vi "Write Channel to Text Log File (Waveform).vi"(6 "Waveform Data":waveform(dbl), 8 "error in (no error)":errorcluster, 9 "Channel Name in":string, 10 "Group Name in":string, 11 "Text Log File in":refnum<class "Text Log File.lvclass">) -> (0 "error out":errorcluster, 3 "Text Log File out":refnum<class "Text Log File.lvclass">)   [LabVIEW 2015, in "Text Log File.lvclass"]
uses:
  Text Log File.lvclass
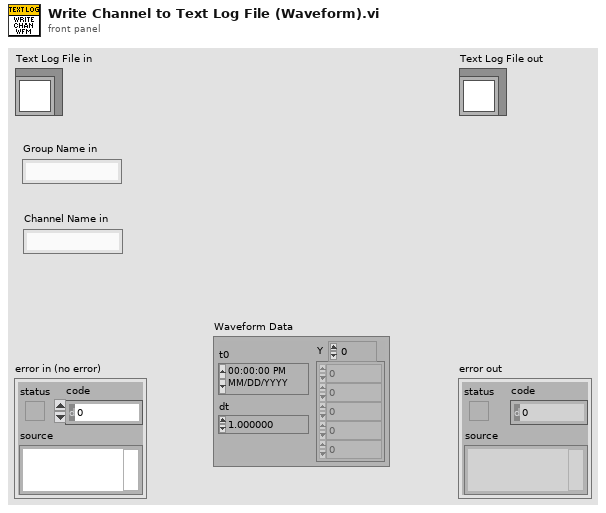
[diagram p1: front panel]
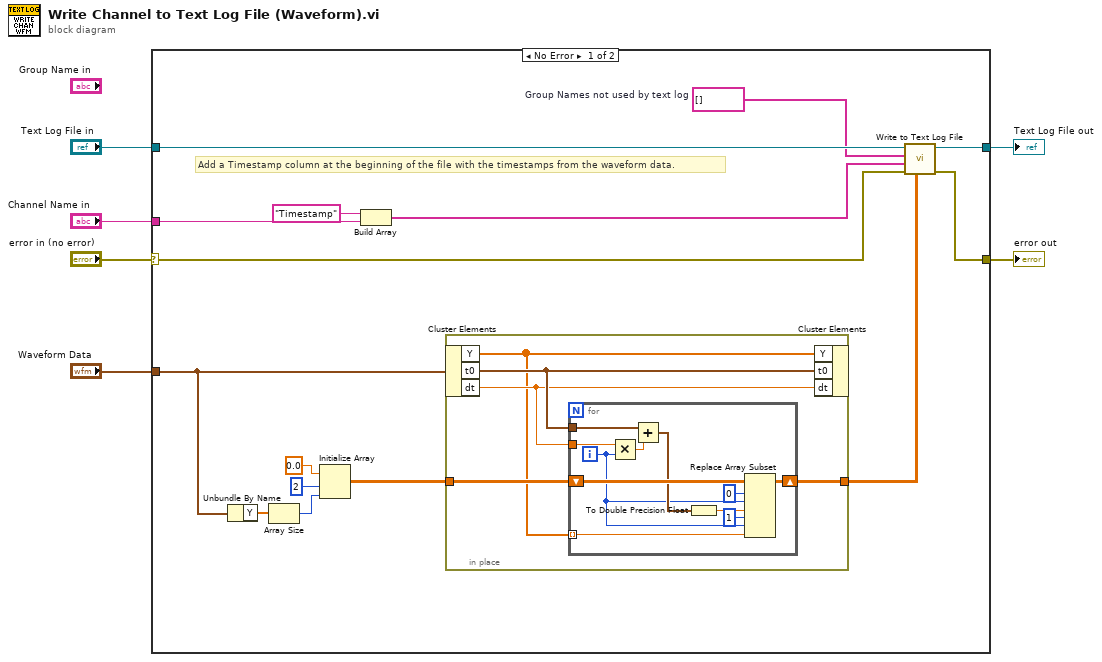
[diagram p0: block diagram]
diagram:
  n1 = case shown="No Error" "error in (no error)" {
    selector: "error in (no error)" -> [w9 w39]
    tunnel: "Waveform Data" -> [w7 _]
    tunnel: "Text Log File in" -> [w17 w38]
    tunnel: [w16 w38] -> w5
    tunnel: "Channel Name in" -> [w15 _]
    tunnel: [w10 w39] -> w4
    frame No Error {
      w13 = string[] []  # Group Names not used by text log
      # "Add a Timestamp column at the beginning of the file with the timestamps from the waveform data."
      n2 = Unbundle By Name(w7) -> ("Y"=w20:dbl[])
      n3 = Array Size(array=w20) -> (size(s)=w19:i32)
      n4 = Initialize Array(0.0, 2 ("dimension size"), w19) -> (w18:dbl[][])
      n5 = Build Array("Timestamp", w15) -> (w12:string[])
      n6 = in-place {
        in-place-border: w18 -> [w24]
        in-place-border: [w23] -> w11
        n7 = in-place-cluster #1(w7) -> ("Y"=w22:dbl[], "t0"=w26:timestamp, "dt"=w25:dbl)
        n8 = for {
          tunnel: w26 -> [w36]
          tunnel: w25 -> [w37]
          shift-right: [w32] -> w23
          shift-left: w24 -> [w34]
          tunnel: w22 -> [w29] mode=indexing
          i -> [w27]
          n9 = Multiply(x=w37, y=w27) -> (x*y=w35:dbl)
          n10 = Add(x=w36, y=w35) -> (x+y=w30:timestamp)
          n11 = To Double Precision Float(number=w30) -> (double precision float=w31:dbl)
          n12 = Replace Array Subset(array=w34, new element #1=w31, index (row) #1=0 ("disabled index (row)"), index (col) #1=w27, new element #2=w29, index (row) #2=1 ("index (row)"), index (col) #2=w27) -> (w32:dbl[][])
        }
        n13 = in-place-cluster #1("Y"=w22, "t0"=w26, "dt"=w25) -> ()  [unwired: 1 out]
      }
      n14 = call "Write to Text Log File.vi"("Data"=w11, "error in (no error)"=w9, "Channel Names in"=w12, "Group Names in"=w13, "Text Log File in"=w17) -> ("error out"=w10:errorcluster, "Text Log File out"=w16:refnum<class "Text Log File.lvclass">)  [unwired: 5 in]
    }
    frame Error {
    }
  }
  "error out" <- w4
  "Text Log File out" <- w5
